vi "test-trapezoid-profile-switch-goal-in-middle-2.vi"() -> (3 "Test Passed":bool)   [LabVIEW 2019]
uses:
  <vilib>/Rock Robotics/WPI/ThirdParty/JAS_Junk/TrajLib/TRAPEZOID_PROFILE_STATE.ctl
  <vilib>/Rock Robotics/WPI/ThirdParty/JAS_Junk/TrajLib/TRAPEZOID_PROFILE.ctl
  <vilib>/Rock Robotics/WPI/ThirdParty/JAS_Junk/TrajLib/TRAPEZOID_PROFILE_CONSTRAINT.ctl
  <vilib>/Rock Robotics/WPI/ThirdParty/JAS_Junk/TrajLib/TrapProfile_ShouldFlipAcceleration.vi
  <vilib>/Rock Robotics/WPI/ThirdParty/JAS_Junk/TrajLib/TrapProfile_Direct.vi
  <vilib>/Rock Robotics/SystemInterfaces/NetworkCommunication/NetComm_UsageReport_report.vi
  <vilib>/Rock Robotics/WPI/ThirdParty/JAS_Junk/TrajLib/Util_LibraryGlobals.vi
  <vilib>/Rock Robotics/WPI/ThirdParty/JAS_Junk/TrajLib/Trajectory_Library.lvlib
panel:
  out "ApproxEquals 2":bool
  out "ApproxEquals":bool
  out "Equal":bool
  out "TRAPEZOID_PROFILE":T1 {"Goal"."Velocity" format="%16_6e"; "Goal"."Position" format="%16_6e"; "Initial"."Velocity" format="%16_6e"; "Initial"."Position" format="%16_6e"; "Constraints"."MaxAcceleration" format="%16_6e"; "Constraints"."MaxVelocity" format="%16_6e"; "EndDecel" format="%16_6e"; "EndFullSpeed" format="%16_6e"; "EndAccel" format="%16_6e"}
  out "State":T3 {"Velocity" format="%16_6e"; "Position" format="%16_6e"}
  out "Waveform Chart":T4(graph)
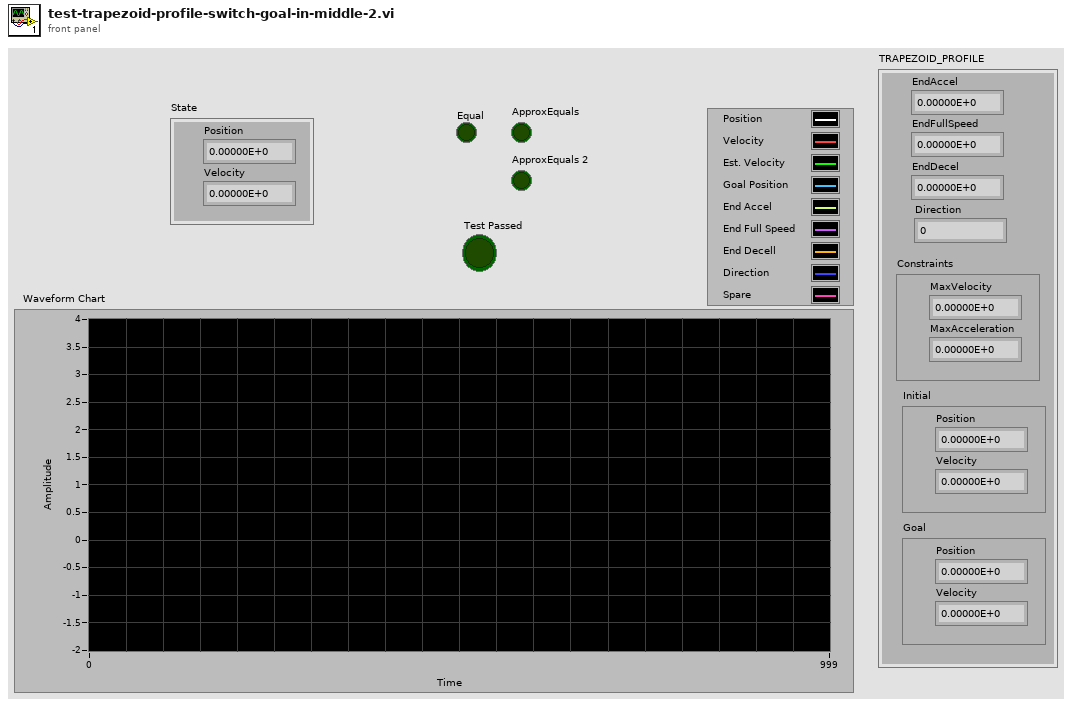
[diagram p1: front panel]
types:
  T1 = typedef "Trajectory_Library.lvlib/TRAPEZOID_PROFILE.ctl" = cluster{"EndAccel":dbl, "EndFullSpeed":dbl, "EndDecel":dbl, "Direction":i32, "Constraints":T2, "Initial":T3, "Goal":T3}
  T2 = typedef "Trajectory_Library.lvlib/TRAPEZOID_PROFILE_CONSTRAINT.ctl" = cluster{"MaxVelocity":dbl, "MaxAcceleration":dbl}
  T3 = typedef "Trajectory_Library.lvlib/TRAPEZOID_PROFILE_STATE.ctl" = cluster{"Position":dbl, "Velocity":dbl}
  T4 = cluster{"Position":dbl, "Velocity":dbl, dbl, "Position":dbl, "EndAccel":dbl, "EndFullSpeed":dbl, "EndDecel":dbl, "Direction":i32, "Position":dbl}
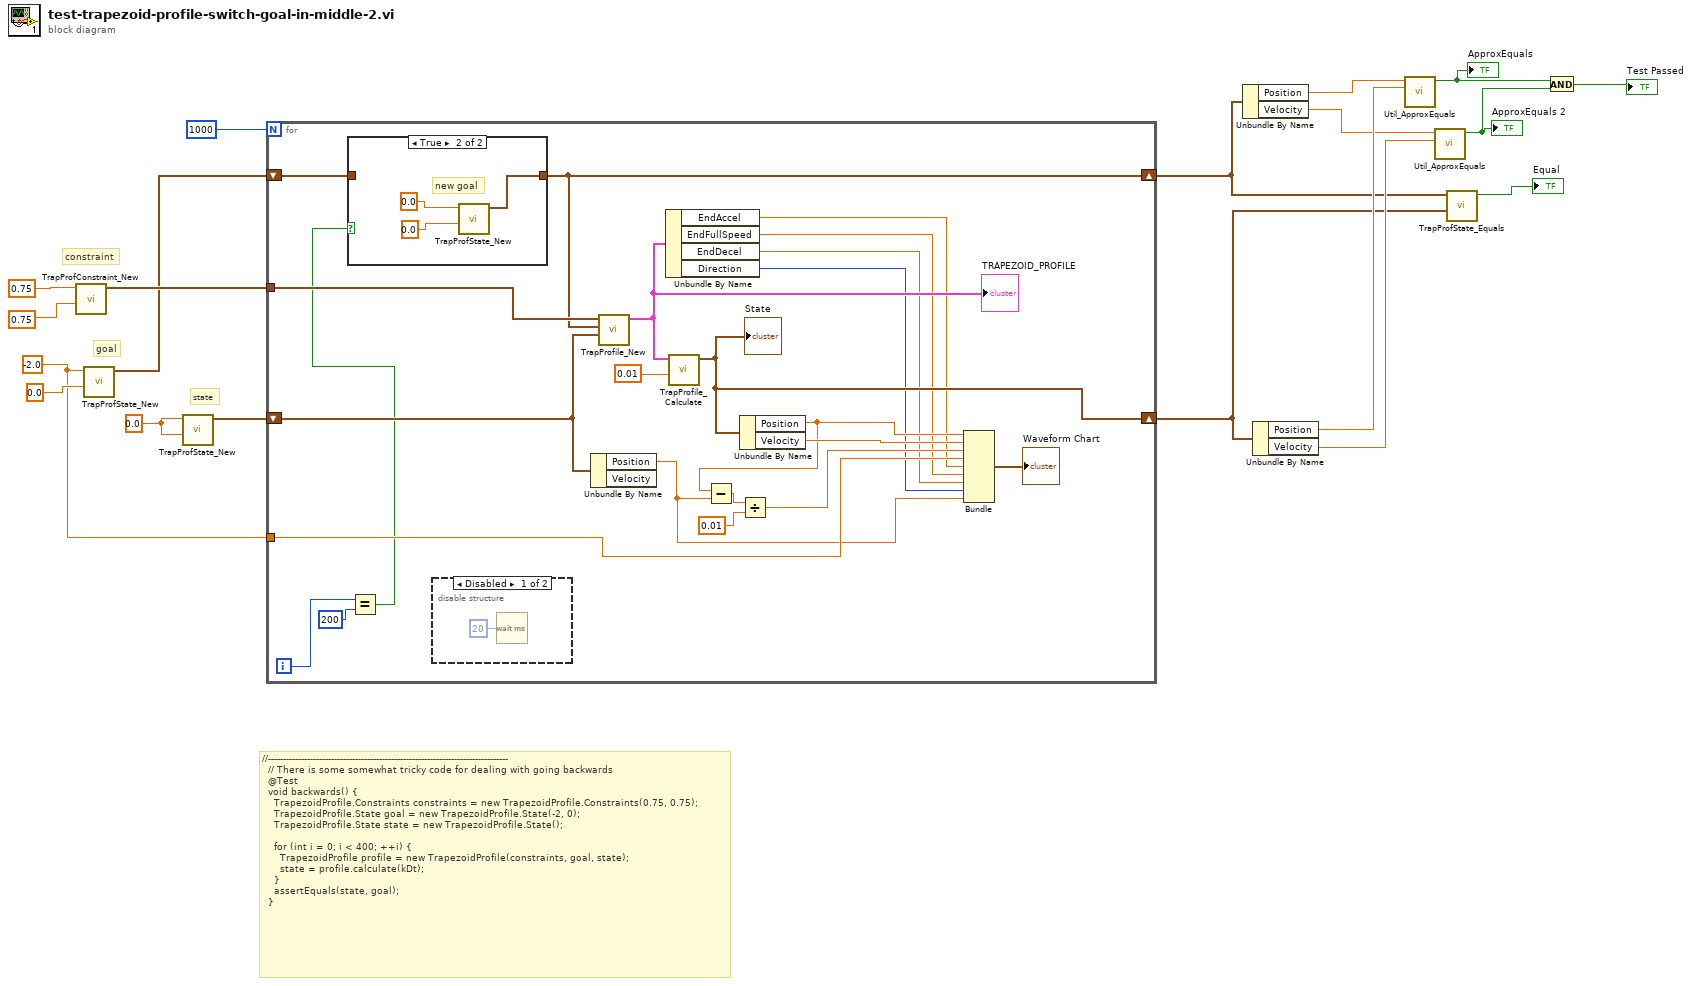
[diagram p0: block diagram]
diagram:
  w15 = 0.0 ("Position")
  w12 = -2.0 ("Position")
  # "state"
  # "//--------------------------------------------------------------------------------\n  // There is some somewhat tricky code for dealing with going backwards\n  @Test\n  void backwards() {\n    TrapezoidProfile.Constraints constraints = new TrapezoidProfile.Constraints(0.75, 0.75);\n    TrapezoidProfile.State goal = new TrapezoidProfile.State(-2, 0);\n    TrapezoidProfile.State state = new TrapezoidProfile.State();\n\n    for (int i = 0; i < 400; ++i) {\n      TrapezoidProfile profile = new TrapezoidProfile(constraints, goal, state);\n      state = profile.calculate(kDt);\n    }\n    assertEquals(state, goal);\n  }"
  # "goal"
  # "constraint"
  n1 = call <vilib>:"TrapProfConstraint_New.vi"("Max Accel"=0.75, "Max Speed (M/S)"=0.75) -> ("TRAPEZOID_PROFILE_CONSTRAINT"=w13:T2)  [unwired: 9 in]
  n2 = call <vilib>:"TrapProfState_New.vi"("Velocity"=0.0, "Position"=w12) -> ("TRAPEZOID_PROFILE_STATE"=w11:T3)  [unwired: 9 in]
  n3 = call <vilib>:"TrapProfState_New.vi"("Velocity"=w15, "Position"=w15) -> ("TRAPEZOID_PROFILE_STATE"=w14:T3)  [unwired: 9 in]
  n4 = for {
    N: 1000 -> [_]
    shift-right: [w33] -> w2
    shift-left: w14 -> [w38]
    tunnel: w12 -> [w32]
    tunnel: w13 -> [w25]
    shift-right: [w20] -> w1
    shift-left: w11 -> [w24]
    i -> [w23]
    n5 = Equal?(x=w23, y=200) -> (x = y?=w21:bool)
    n6 = case shown="True" w21 {
      tunnel: w24 -> [w43 _]
      tunnel: [w43 w44] -> w20
      frame False {
      }
      frame True {
        # "new goal"
        n7 = call <vilib>:"TrapProfState_New.vi"("Velocity"=0.0, "Position"=0.0) -> ("TRAPEZOID_PROFILE_STATE"=w44:T3)  [unwired: 9 in]
      }
    }
    n8 = disable-structure shown="Disabled" {
      frame Disabled {
        n9 = Wait (ms)(milliseconds to wait=u32 20) -> ()  [unwired: 1 out]
      }
      frame Enabled {
      }
    }
    n10 = Unbundle By Name(w38) -> ("Position"=w26:dbl)  [unwired: 1 out]
    n11 = call <vilib>:"TrapProfile_New.vi"("Initial"=w38, "Goal"=w20, "Constraints"=w25) -> ("TRAPEZOID_PROFILE"=w31:T1)  [unwired: 8 in]
    "TRAPEZOID_PROFILE" <- w31
    n12 = Unbundle By Name(w31) -> ("EndAccel"=w30:dbl, "EndFullSpeed"=w29:dbl, "EndDecel"=w28:dbl, "Direction"=w27:i32)
    n13 = call <vilib>:"TrapProfile_Calculate.vi"("Time"=0.01, "TRAPEZOID_PROFILE"=w31) -> ("State"=w33:T3)  [unwired: 9 in]
    "State" <- w33
    n14 = Unbundle By Name(w33) -> ("Position"=w37:dbl, "Velocity"=w40:dbl)
    n15 = Subtract(x=w37, y=w26) -> (x-y=w36:dbl)
    n16 = Divide(x=w36, y=0.01) -> (x/y=w34:dbl)
    n17 = Bundle("Position"=w37, "Velocity"=w40, w34, "Position"=w32, "EndAccel"=w30, "EndFullSpeed"=w29, "EndDecel"=w28, "Direction"=w27, "Position"=w26) -> (→"Waveform Chart":T4)  [unwired: 1 in]
  }
  n18 = Unbundle By Name(w1) -> ("Position"=w10:dbl, "Velocity"=w8:dbl)
  n19 = Unbundle By Name(w2) -> ("Position"=w9:dbl, "Velocity"=w6:dbl)
  n20 = call <vilib>:"Util_ApproxEquals.vi"("Value 2"=w9, "Value 1"=w10) -> ("ApproxEquals"=w4:bool)  [unwired: 9 in]
  "ApproxEquals" <- w4
  n21 = call <vilib>:"Util_ApproxEquals.vi"("Value 2"=w6, "Value 1"=w8) -> ("ApproxEquals"=w3:bool)  [unwired: 9 in]
  "ApproxEquals 2" <- w3
  n22 = call <vilib>:"TrapProfState_Equals.vi"("TRAPEZOID_PROFILE_STATE 2"=w2, "TRAPEZOID_PROFILE_STATE"=w1) -> ("Equal"=→"Equal":bool)  [unwired: 9 in]
  n23 = And(x=w4, y=w3) -> (x .and. y?=→"Test Passed":bool)
